vi "shipping.vi"() -> ()   [LabVIEW 2012]
uses:
  <vilib>/Utility/NIReport.llb/NI_report.lvclass
  Global1.vi
  <vilib>/addons/database/Connection.llb/DB Tools Open Connec (Path).vi
  <vilib>/addons/_office/excel.llb/Excel Get Data (str).vi
  <vilib>/Utility/NIReport.llb/Excel/NI_Excel.lvclass
  <vilib>/addons/_office/NI_ReportGenerationToolkit.lvlib
  <vilib>/addons/database/NI_Database_API.lvlib
panel:
  out "error out 2":errorcluster
  out "x+y":i32
  out "row":i32
  out "String 3":string
  out "String 2":string
  out "String":string
  out "data":string
  out "error out":errorcluster
  in  "start (0, 0)":cluster{"start row":i32, "start column":i32}
  out "error out 4":errorcluster
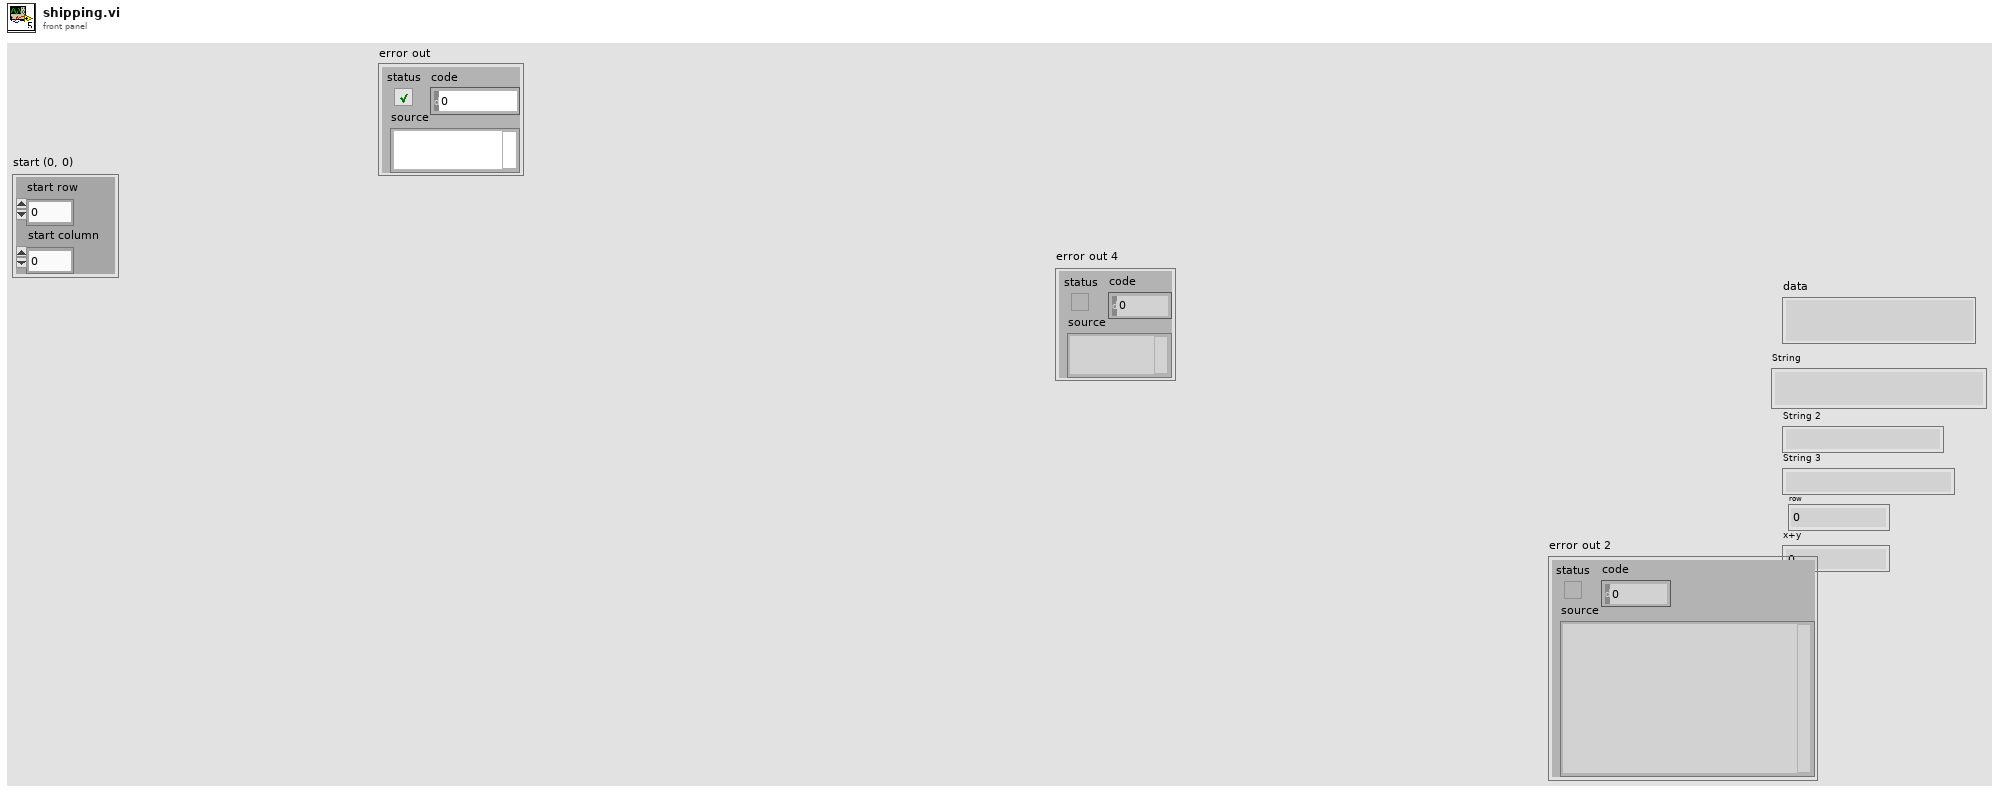
[diagram p1: front panel]
types:
  T1 = enum16{"Standard Report", "HTML", "Word", "Excel"}
  T2 = typedef "NI_Database_API.lvlib/Conn ObjectReference.ctl" = refnum<k1>
  T3 = cluster{"on/off":bool, "weight":i32, "color":u32}
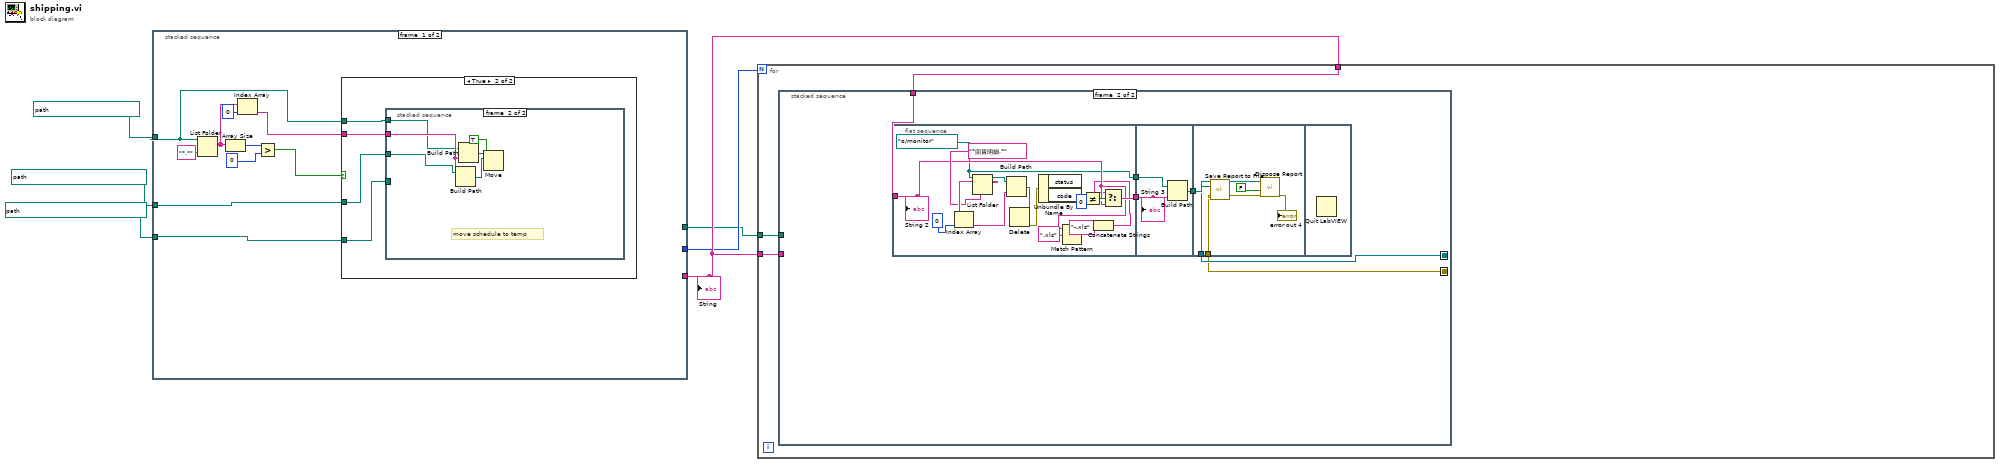
[diagram p0: block diagram]
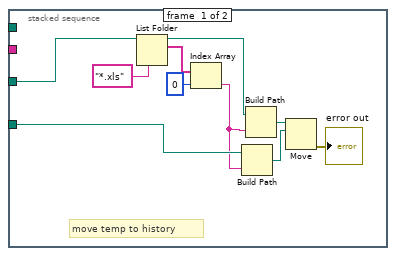
[diagram p3: hidden frame]
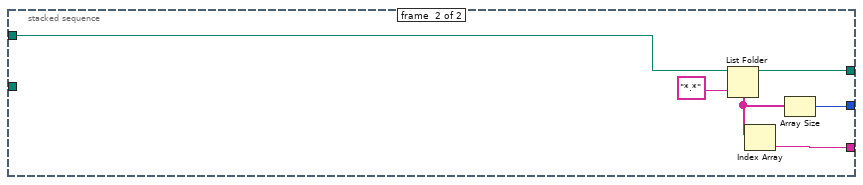
[diagram p4: hidden frame]
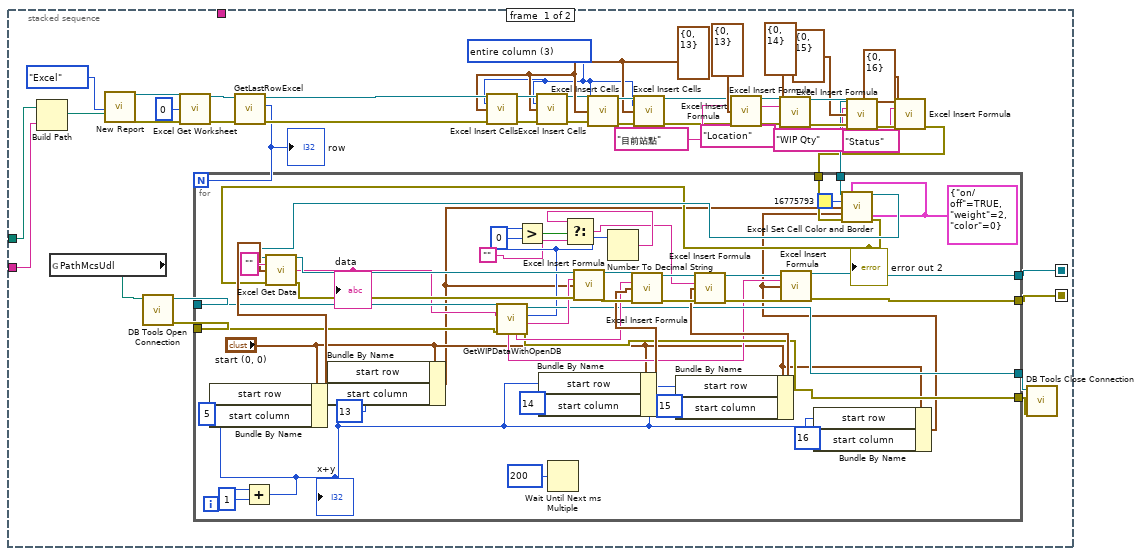
[diagram p5: hidden frame]
diagram:
  n1 = stacked-sequence {
    tunnel: path "o:/monitor/回貨明細/temp" ("path") -> [w8 w41]
    tunnel: [_ w40] -> w2
    tunnel: [_ w39] -> w1
    tunnel: [_ w37] -> w3
    tunnel: path "o:/monitor/回貨明細" ("path") -> [w10 _]
    tunnel: path "o:/monitor/回貨明細/history" ("path") -> [w9 _]
    frame #0 {
      n2 = List Folder(path=w10, pattern="*.*") -> (filenames=w13:string[])  [unwired: 2 in, 3 out]
      n3 = Array Size(array=w13) -> (size(s)=w15:i32)
      n4 = Index Array(array=w13, index=0) -> (element=w12:string)
      n5 = Greater?(x=w15, y=0) -> (0:w7:bool)
      n6 = case shown="True" w7 {
        tunnel: w8 -> [_ w20]
        tunnel: w9 -> [_ w19]
        tunnel: w10 -> [_ w18]
        tunnel: w12 -> [_ w17]
        frame False {
        }
        frame True {
          n7 = stacked-sequence {
            tunnel: w20 -> [w26 w32]
            tunnel: w19 -> [w29 _]
            tunnel: w18 -> [_ w33]
            tunnel: w17 -> [_ w34]
            frame #0 {
              # "move temp to history"
              n8 = List Folder(path=w26, pattern="*.xls") -> (path out=w24:path, filenames=w23:string[])  [unwired: 2 in, 2 out]
              n9 = Index Array(array=w23, index=0) -> (element=w21:string)
              n10 = Build Path(base path=w29, name or relative path=w21) -> (appended path=w28:path)
              n11 = Build Path(base path=w24, name or relative path=w21) -> (appended path=w30:path)
              n12 = Move(source path=w30, 10:w28) -> (error out=→"error out":errorcluster)  [unwired: 3 in, 2 out]
            }
            frame #1 {
              # "move schedule to temp"
              n13 = Build Path(base path=w32, name or relative path=w34) -> (appended path=w35:path)
              n14 = Build Path(base path=w33, name or relative path=w34) -> (appended path=w36:path)
              n15 = Move(source path=w36, 9:TRUE ("overwrite (F)"), 10:w35) -> ()  [unwired: 2 in, 3 out]
            }
          }
        }
      }
    }
    frame #1 {
      n16 = List Folder(path=w41, pattern="*.*") -> (path out=w39:path, filenames=w38:string[])  [unwired: 2 in, 2 out]
      n17 = Index Array(array=w38) -> (element=w37:string)  [unwired: 1 in]
      n18 = Array Size(array=w38) -> (size(s)=w40:i32)
    }
  }
  "String" <- w3
  n19 = for {
    N: w2 -> [_]
    tunnel: w1 -> [w45]
    tunnel: w3 -> [w44]
    tunnel: w3 -> [w43]
    n20 = stacked-sequence {
      seq-local: [w67 _] -> [_ w137]
      seq-local: [w53 _] -> [_ w138]
      tunnel: w45 -> [w90 _]
      tunnel: w44 -> [w89 _]
      tunnel: w43 -> [_ w140]
      frame #0 {
        w60 = cluster{"row":i32, "column":i32} {"row"=0, "column"=13} ("start (0, 0)")
        w57 = u16 3 items=["shift cells right", "shift cells down", "entire row", "entire column"] ("mode (entire row)")
        n21 = Build Path(base path=w90, name or relative path=w89) -> (appended path=w88:path)
        n22 = global read "Global1.vi" "PathMcsUdl"() -> (w80:path)
        n23 = call <vilib>:"New Report.vi"("report type"=T1."Excel" ("Report Type"), "template (empty)"=w88) -> ("report out"=w86:refnum<class "NI_report.lvclass">, "error out"=w85:errorcluster)  [unwired: 12 in]
        n24 = call-poly <vilib>:"DB Tools Open Connection.vi"("connection information"=w80) -> ("error out"=w78:errorcluster, "connection reference"=w79:T2)  [unwired: 7 in]
        n25 = call <vilib>:"Excel Get Worksheet.vi"("report in"=w86, "worksheet index (0)"=0, "error in (no error)"=w85) -> ("report out"=w66:refnum<class "NI_report.lvclass">, "error out"=w65:errorcluster)  [unwired: 11 in]
        n26 = call "GetLastRowExcel.vi"("error in (no error)"=w65, "report in"=w66) -> ("error out"=w64:errorcluster, "row"=w48:i32, "report out"=w63:refnum<class "NI_report.lvclass">)  [unwired: 7 in]
        "row" <- w48
        n27 = call <vilib>:"Excel Insert Cells.vi"("report in"=w63, "mode (entire row)"=w57, "start (0, 0)"=w60, "error in (no error)"=w64) -> ("report out"=w62:refnum<class "NI_report.lvclass">, "error out"=w61:errorcluster)  [unwired: 10 in]
        n28 = call <vilib>:"Excel Insert Cells.vi"("report in"=w62, "mode (entire row)"=w57, "start (0, 0)"=w60, "error in (no error)"=w61) -> ("report out"=w59:refnum<class "NI_report.lvclass">, "error out"=w58:errorcluster)  [unwired: 10 in]
        n29 = call <vilib>:"Excel Insert Cells.vi"("report in"=w59, "mode (entire row)"=w57, "start (0, 0)"=w60, "error in (no error)"=w58) -> ("report out"=w84:refnum<class "NI_report.lvclass">, "error out"=w83:errorcluster)  [unwired: 10 in]
        n30 = call <vilib>:"Excel Insert Cells.vi"("report in"=w84, "mode (entire row)"=w57, "start (0, 0)"=w60, "error in (no error)"=w83) -> ("report out"=w50:refnum<class "NI_report.lvclass">, "error out"=w49:errorcluster)  [unwired: 10 in]
        n31 = call <vilib>:"Excel Insert Formula.vi"("report in"=w50, "formula"="目前站點", "start (0, 0)"=cluster{"row":i32, "column":i32} {"row"=0, "column"=13}, "error in (no error)"=w49) -> ("report out"=w77:refnum<class "NI_report.lvclass">, "error out"=w75:errorcluster)  [unwired: 10 in]
        n32 = call <vilib>:"Excel Insert Formula.vi"("report in"=w77, "formula"="Location", "start (0, 0)"=cluster{"row":i32, "column":i32} {"row"=0, "column"=14}, "error in (no error)"=w75) -> ("report out"=w76:refnum<class "NI_report.lvclass">, "error out"=w74:errorcluster)  [unwired: 10 in]
        n33 = call <vilib>:"Excel Insert Formula.vi"("report in"=w76, "formula"="WIP Qty", "start (0, 0)"=cluster{"row":i32, "column":i32} {"row"=0, "column"=15}, "error in (no error)"=w74) -> ("report out"=w56:refnum<class "NI_report.lvclass">, "error out"=w55:errorcluster)  [unwired: 10 in]
        n34 = call <vilib>:"Excel Insert Formula.vi"("report in"=w56, "formula"="Status", "start (0, 0)"=cluster{"row":i32, "column":i32} {"row"=0, "column"=16}, "error in (no error)"=w55) -> ("report out"=w47:refnum<class "NI_report.lvclass">, "error out"=w46:errorcluster)  [unwired: 10 in]
        n35 = for {
          N: w48 -> [_]
          tunnel: [w100] -> w67
          tunnel: [w120] -> w82
          tunnel: [w119] -> w81
          tunnel: w79 -> [w118]
          tunnel: w78 -> [w117]
          tunnel: [w101] -> w53
          tunnel: w47 -> [w97]
          tunnel: w46 -> [w96]
          i -> [w110]
          w95 = T3 {"on/off"=TRUE, "weight"=2, "color"=0} ("outside border")
          n36 = Add(x=w110, y=1) -> (x+y=w104:i32)
          "x+y" <- w104
          n37 = Bundle By Name(cluster="start (0, 0)", "start row"=w104, "start column"=5) -> (w132:cluster{"start row":i32, "start column":i32})
          n38 = Bundle By Name(cluster="start (0, 0)", "start row"=w104, "start column"=13) -> (w93:cluster{"start row":i32, "start column":i32})
          n39 = Bundle By Name(cluster="start (0, 0)", "start row"=w104, "start column"=14) -> (w123:cluster{"start row":i32, "start column":i32})
          n40 = Wait Until Next ms Multiple(millisecond multiple=u32 200) -> ()  [unwired: 1 out]
          n41 = Bundle By Name(cluster="start (0, 0)", "start row"=w104, "start column"=15) -> (w124:cluster{"start row":i32, "start column":i32})
          n42 = Bundle By Name(cluster="start (0, 0)", "start row"=w104, "start column"=16) -> (w92:cluster{"start row":i32, "start column":i32})
          n43 = call <vilib>:"Excel Set Cell Color and Border.vi"("report in"=w97, "inside border"=w95, "outside border"=w95, "background color (w)"=u32 16775793, "start (-1, -1)"=w93, "end (-1, -1)"=w92, "error in (no error)"=w96) -> ("report out"=w99:refnum<class "NI_report.lvclass">, "error out"=w98:errorcluster)  [unwired: 7 in]
          "error out 2" <- w98
          n44 = call-poly <vilib>:"Excel Get Data.vi"("report in"=w99, "data type"="", "start (0, 0)"=w132, "error in (no error)"=w98) -> ("report out"=w135:refnum<class "NI_report.lvclass">, "data"=w102:string, "error out"=w134:errorcluster)  [unwired: 9 in]
          "data" <- w102
          n45 = call "GetWIPDataWithOpenDB.vi"("error in (no error)"=w117, "Lotno"=w102, "connection reference"=w118) -> ("error out"=w119:errorcluster, "step"=w122:string, "data"=w115:i32, "connection reference 2"=w120:T2, "location"=w121:string, "status"=w105:string)  [unwired: 3 in]
          n46 = Greater?(x=w115, y=0) -> (0:w113:bool)
          n47 = call <vilib>:"Excel Insert Formula.vi"("report in"=w135, "formula"=w122, "start (0, 0)"=w93, "error in (no error)"=w134) -> ("report out"=w128:refnum<class "NI_report.lvclass">, "error out"=w125:errorcluster)  [unwired: 10 in]
          n48 = Number To Decimal String(number=w115) -> (decimal integer string=w114:string)  [unwired: 1 in]
          n49 = Select(t=w114, s=w113, f="") -> (s? t:f=w111:string)
          n50 = call <vilib>:"Excel Insert Formula.vi"("report in"=w128, "formula"=w121, "start (0, 0)"=w123, "error in (no error)"=w125) -> ("report out"=w127:refnum<class "NI_report.lvclass">, "error out"=w126:errorcluster)  [unwired: 10 in]
          n51 = call <vilib>:"Excel Insert Formula.vi"("report in"=w127, "formula"=w111, "start (0, 0)"=w124, "error in (no error)"=w126) -> ("report out"=w107:refnum<class "NI_report.lvclass">, "error out"=w106:errorcluster)  [unwired: 10 in]
          n52 = call <vilib>:"Excel Insert Formula.vi"("report in"=w107, "formula"=w105, "start (0, 0)"=w92, "error in (no error)"=w106) -> ("report out"=w101:refnum<class "NI_report.lvclass">, "error out"=w100:errorcluster)  [unwired: 10 in]
        }
        n53 = call <vilib>:"DB Tools Close Connection.vi"("error in (no error)"=w81, "connection reference"=w82) -> ()  [unwired: 5 in, 1 out]
      }
      frame #1 {
        n54 = flat-sequence {
          tunnel: [w143] -> w142
          tunnel: w140 -> [w145]
          tunnel: [w146] -> w141
          tunnel: w142 -> [w162]
          tunnel: w141 -> [w161]
          tunnel: [w160] -> w139
          tunnel: w139 -> [w165]
          tunnel: w138 -> [w164]
          tunnel: w137 -> [w163]
          frame #0 {
            w143 = path "o:/monitor" ("base path")
            n55 = List Folder(path=w143, pattern="*回貨明細.*") -> (path out=w157:path, filenames=w159:string[])  [unwired: 2 in, 2 out]
            n56 = Index Array(array=w159, index=0) -> (element=w156:string)
            n57 = Build Path(base path=w157, name or relative path=w156) -> (appended path=w154:path)
            n58 = Delete(path (use dialog)=w154) -> (error out=w153:errorcluster)  [unwired: 4 in, 2 out]
            n59 = Unbundle By Name(w153) -> ("code"=w152:i32)  [unwired: 1 out]
            n60 = Match Pattern(string=w145, regular expression=".xls") -> (match substring=w148:string)  [unwired: 1 in, 3 out]
            n61 = Not Equal?(x=w152, y=0) -> (x != y?=w150:bool)
            n62 = Concatenate Strings(w148, "-.xls" ("string")) -> (w144:string)
            n63 = Select(t=w144, s=w150, f=w145) -> (s? t:f=w146:string)
            "String 2" <- w145
          }
          frame #1 {
            n64 = Build Path(base path=w162, name or relative path=w161) -> (appended path=w160:path)
            "String 3" <- w161
          }
          frame #2 {
            n65 = call-dynamic "Save Report to File.vi"("report in"=w164, "report file path"=w165, "error in (no error)"=w163) -> ("report out"=w166:refnum<class "NI_report.lvclass">, "error out"=w167:errorcluster)  [unwired: 11 in]
            n66 = call-dynamic "Dispose Report.vi"("report in"=w166, "save changes? (F)"=FALSE, "error in (no error)"=w167) -> ("error out"=→"error out 4":errorcluster)  [unwired: 12 in]
          }
          frame #3 {
            n67 = Quit LabVIEW() -> ()  [unwired: 1 in]
          }
        }
      }
    }
  }
